vi "Count.vi"(8 "error in (no error)":errorcluster, 11 "Dictionary in":refnum<class "Dictionary.lvclass">) -> (0 "error out":errorcluster, 2 "Size":i32, 3 "Dictionary out":refnum<class "Dictionary.lvclass">)   [LabVIEW 2018, in "Application.lvlib" / "Dictionary.lvclass"]
uses:
  Dictionary.lvclass
  Dictionary.lvclass/Dictionary.ctl
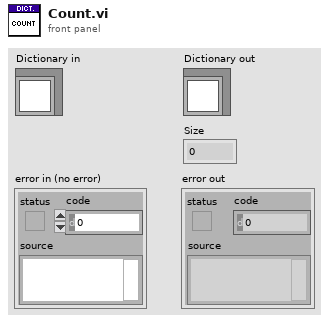
[diagram p1: front panel]
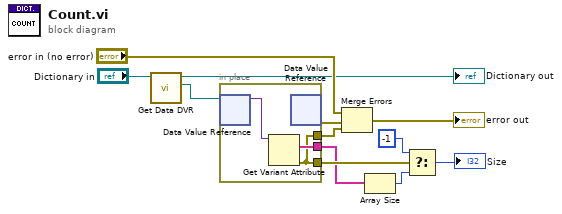
[diagram p0: block diagram]
diagram:
  n1 = call "Get Data DVR.vi"("Dictionary in"="Dictionary in") -> ("Data DVR"=w6:refnum<data-value>, "Dictionary out"=→"Dictionary out":refnum<class "Dictionary.lvclass">)  [unwired: 8 in, 1 out]
  n2 = in-place {
    in-place-border: [w14] -> w1
    in-place-border: [w13] -> w9
    in-place-border: [w13] -> w5
    n3 = in-place-dvr #1(w6) -> (w15:variant)  [unwired: 1 out]
    n4 = Get Variant Attribute(Variant=w15) -> (names=w14:string[], error out=w13:errorcluster)  [unwired: 3 in, 2 out]
    n5 = in-place-dvr #1() -> (w11:errorcluster)  [unwired: 1 in, 1 out]
  }
  n6 = Merge Errors("error in (no error)", w11, w9) -> (→"error out":errorcluster)
  n7 = Array Size(array=w1) -> (size(s)=w4:i32)
  n8 = Select(t=-1, s=w5, f=w4) -> (s? t:f=→"Size":i32)
